vi "Disabled.vi"(7 "Robot Mode":T2=enum."Teleop Disabled", 10 "Match Info":T1={"Autonomous Elapsed Seconds"=0.0, "TeleOp Elapsed Seconds"=133.578, "Disabled Elapsed Seconds"=12.599, "Visited Autonomous"=FALSE, "Visited TeleOp"=TRUE, "Visited Disabled"=TRUE, "Autonomous Settings"={"Autonomous Style"=enum."Independent", "VI Refnum"=refnum}}, 11 "Call Context":T3=enum."Stop") -> ()   [LabVIEW 2012]
doc: "This VI is called each time a disabled packet is received from the DS. It is often used to prepare for the next robot mode, to calibrate sensors, etc."
uses:
  <vilib>/Rock Robotics/WPI/DriverStation/WPI_DriverStationDerivedRobotMode.ctl
  <vilib>/Rock Robotics/WPI/DriverStation/WPI_DriverStationRobotMode.ctl
  <vilib>/Rock Robotics/WPI/DriverStation/WPI_DriverStationMatch Info.ctl
  <vilib>/Rock Robotics/WPI/Solenoid/WPI_SolenoidValue.ctl
  Robot Global Data.vi
  <vilib>/Rock Robotics/WPI/Solenoid/WPI_SolenoidSetEnum.vi
panel:
  in  "Pitch Calib. Factor\nOLD ROBOT":dbl=-6.5
  in  "Encoder Codes\n Per Foot OLD Robot":u16=300
  in  "Feet/Second\n at FT OLD Robot":dbl=10.0
  in  "Encoder Codes\n Per Foot":u16=907
  in  "Feet/Second\n at Full Throttle":dbl=15.0
  in  "Pitch Calib. Factor\nNEW ROBOT":dbl=-1.7
  out "Loop Time":u32=23
  # "OLD"
  # "NEW"
  # "15"
  # "15   2011 Robot"
  # "907"
  # "300   2011 Robot"
  # "-0.5"
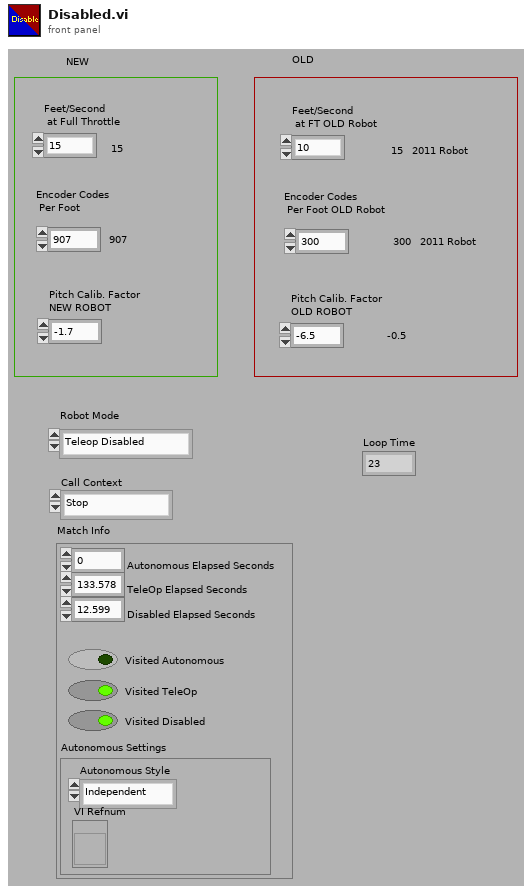
[diagram p1: front panel]
types:
  T1 = typedef "WPI_DriverStationMatch Info.ctl" = cluster{"Autonomous Elapsed Seconds":dbl, "TeleOp Elapsed Seconds":dbl, "Disabled Elapsed Seconds":dbl, "Visited Autonomous":bool, "Visited TeleOp":bool, "Visited Disabled":bool, "Autonomous Settings":cluster{"Autonomous Style":enum16{"Iterative", "Independent"}, "VI Refnum":refnum<vi>}}
  T2 = typedef "WPI_DriverStationRobotMode.ctl" = enum16{"Autonomous Disabled", "Autonomous Enabled", "Teleop Disabled", "Teleop Enabled", "Timeout", "Finish"}
  T3 = typedef "WPI_DriverStationDerivedRobotMode.ctl" = enum16{"Init", "Execute", "Stop"}
  T4 = typedef "WPI_SolenoidValue.ctl" = enum16{"Off", "On", "Forward", "Reverse"}
  T5 = typedef "WPI_SolenoidDevRef.ctl" = cluster{"DevStatus":errorcluster, "Solenoid Module":T6, "Forward Solenoid Channel":T7, "Reverse Solenoid Channel":T7}
  T6 = typedef "FPGA_TypedefSolenoidModule.ctl" = enum16{"Solenoid Module 1", "Solenoid Module 2"}
  T7 = typedef "WPI_SolenoidChannel.ctl" = enum8{"Solenoid 1", "Solenoid 2", "Solenoid 3", "Solenoid 4", "Solenoid 5", "Solenoid 6", "Solenoid 7", "Solenoid 8", "Invalid"}
  T8 = typedef "WPI_CounterDevRef.ctl" = cluster{"DevStatus":errorcluster, "CntIndex":T9}
  T9 = typedef "FPGA_CounterCtrSystemIndex.ctl" = enum8{"Ctr 0", "Ctr 1", "Ctr 2", "Ctr 3", "Ctr 4", "Ctr 5", "Ctr 6", "Ctr 7", "Invalid"}
  T10 = typedef "WPI_DigitalInputDevRef.ctl" = cluster{"DevStatus":errorcluster, "DIO Channel":T11, "Digital Module":T12}
  T11 = typedef "FPGA_DIOChannel.ctl" = enum8{"DIO 1", "DIO 2", "DIO 3", "DIO 4", "DIO 5", "DIO 6", "DIO 7", "DIO 8", "DIO 9", "DIO 10", "DIO 11", "DIO 12", "DIO 13", "DIO 14", "Invalid"}
  T12 = typedef "FPGA_TypedefDigitalModule.ctl" = enum16{"Digital Module 1", "Digital Module 2"}
  T13 = typedef "WPI_EncoderDevRef.ctl" = cluster{"DevStatus":errorcluster, "EncoderIndex":T14, "CounterIndex":T9, "DistancePerCount":dbl, "Decoding Type":T15}
  T14 = typedef "FPGA_EncoderIdx.ctl" = enum8{"Enc 0", "Enc 1", "Enc 2", "Enc 3", "Invalid"}
  T15 = typedef "WPI_EncoderType.ctl" = enum16{"1x", "2x", "4x"}
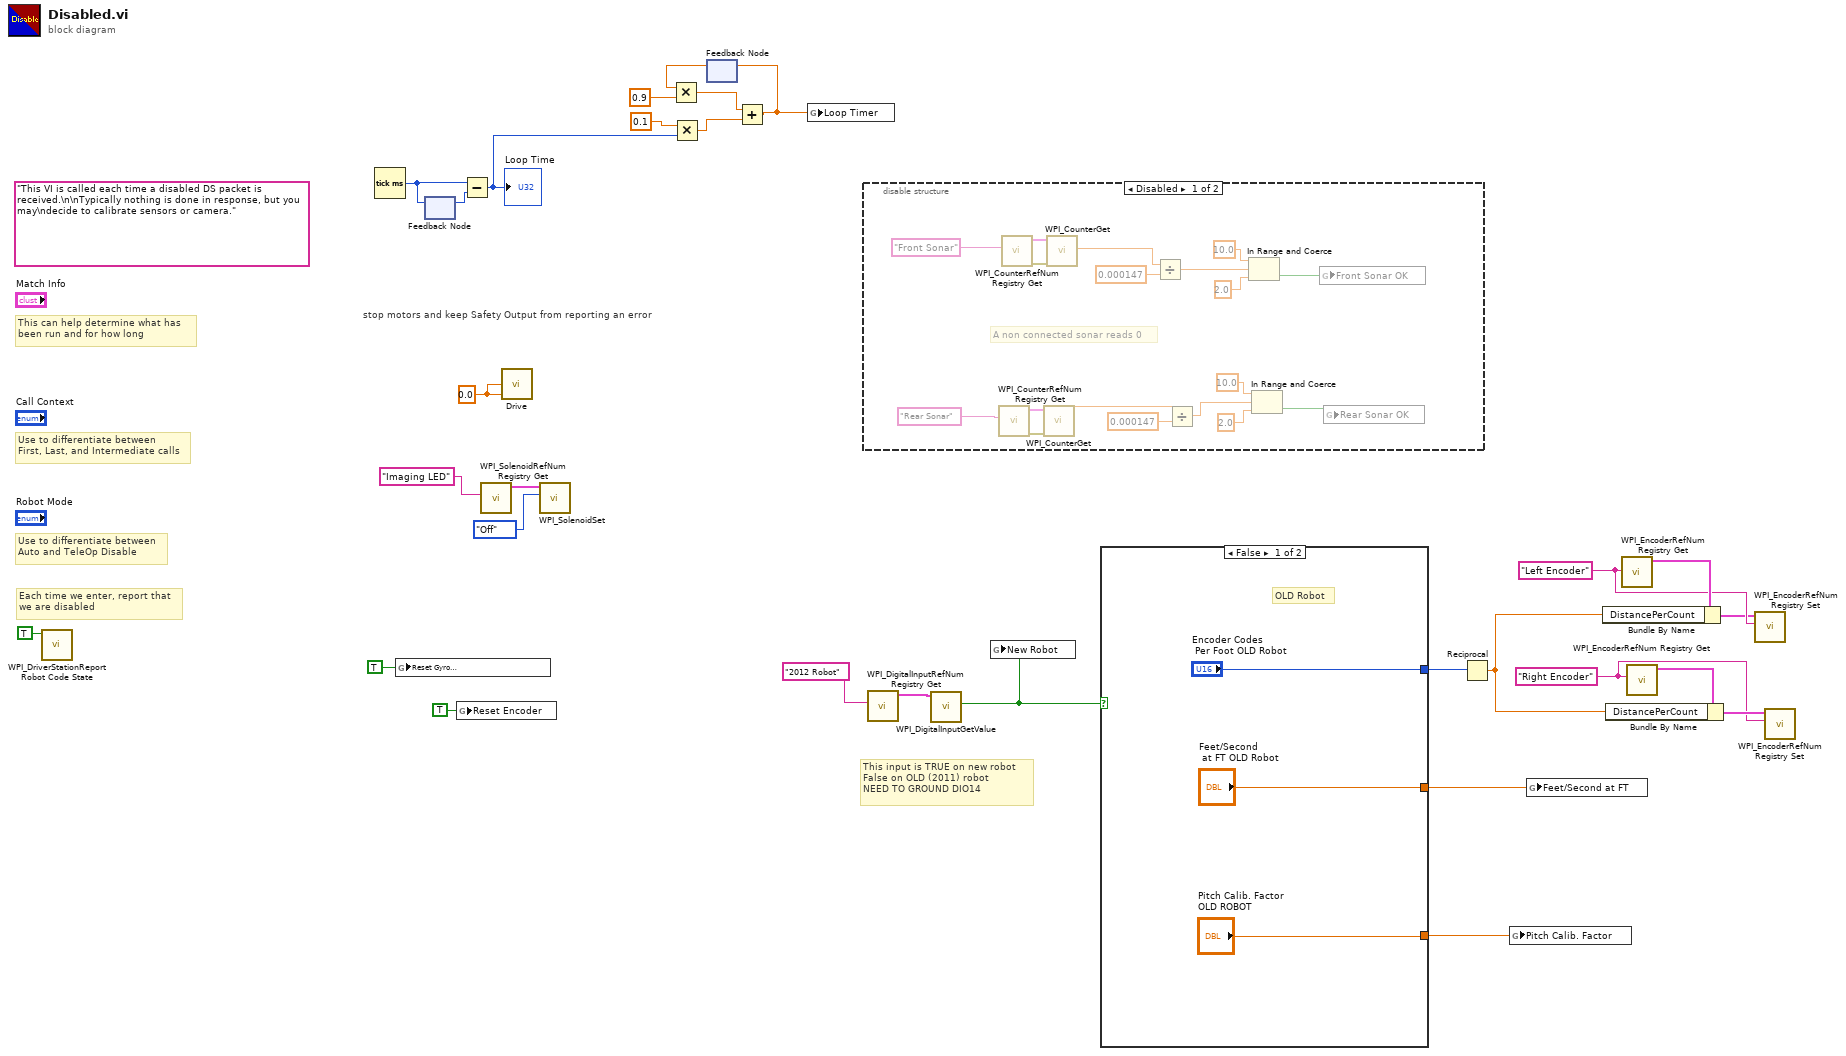
[diagram p0: block diagram]
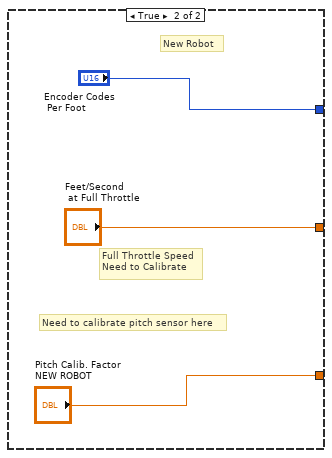
[diagram p3: hidden frame]
diagram:
  w3 = 0.0 ("Right Motor IN")
  w16 = "Right Encoder" ("refnum name")
  w21 = "Left Encoder" ("refnum name")
  (unwired) "This VI is called each time a disabled DS packet is received.\n\nTypically nothing is done in response, but you may\ndecide to calibrate sensors or camera."
  # "This input is TRUE on new robot\nFalse on OLD (2011) robot \nNEED TO GROUND DIO14"
  # "stop motors and keep Safety Output from reporting an error"
  # "Each time we enter, report that\nwe are disabled"
  # "Use to differentiate between\nFirst, Last, and Intermediate calls"
  # "This can help determine what has\nbeen run and for how long"
  # "Use to differentiate between\nAuto and TeleOp Disable"
  n1 = call <vilib>:"WPI_DriverStationReport Robot Code State.vi"("Disabled"=TRUE ("Autonomous")) -> ()  [unwired: 10 in, 1 out]
  n2 = Tick Count (ms)() -> (millisecond timer value=w27:u32)
  n3 = global write "Robot Global Data.vi" "Reset Gyro\nZero Position"(TRUE ("Reset Gyro\nZero Position")) -> ()
  n4 = feedback #1() -> (w28:u32)  [unwired: 1 in]
  n5 = feedback-in #1(w27) -> ()
  n6 = global write "Robot Global Data.vi" "Reset Encoder"(TRUE ("Reset Encoder")) -> ()
  n7 = Subtract(x=w27, y=w28) -> (x-y=w9:u32)
  "Loop Time" <- w9
  n8 = call <vilib>:"WPI_SolenoidRefNum Registry Get.vi"("refnum name"="Imaging LED") -> ("SolenoidDevRef"=w6:T5)  [unwired: 9 in, 1 out]
  n9 = call "Drive.vi"("Right Motor IN"=w3, "Left Motor IN"=w3) -> ()  [unwired: 3 in, 1 out]
  n10 = call-poly <vilib>:"WPI_SolenoidSet.vi"("Value"=WPI_SolenoidValue."Off", "SolenoidDevRef"=w6) -> ()  [unwired: 8 in, 2 out]
  n11 = Multiply(x=0.1, y=w9) -> (x*y=w11:dbl)
  n12 = feedback #2() -> (w13:dbl)  [unwired: 1 in]
  n13 = Multiply(x=w13, y=0.9) -> (x*y=w12:dbl)
  n14 = Add(x=w12, y=w11) -> (x+y=w15:dbl)
  n15 = feedback-in #2(w15) -> ()
  n16 = global write "Robot Global Data.vi" "Loop Timer"(w15) -> ()
  n17 = disable-structure shown="Disabled" {
    frame Disabled {
      # "A non connected sonar reads 0"
      n18 = call <vilib>:"WPI_CounterRefNum Registry Get.vi"("refnum name"="Rear Sonar") -> ("error out"=w43:errorcluster, "CounterDevRef"=w42:T8)  [unwired: 9 in]
      n19 = call <vilib>:"WPI_CounterRefNum Registry Get.vi"("refnum name"="Front Sonar") -> ("error out"=w47:errorcluster, "CounterDevRef"=w46:T8)  [unwired: 9 in]
      n20 = call <vilib>:"WPI_CounterGet.vi"("error in (no error)"=w43, "CounterDevRef in"=w42) -> ("Period (sec)"=w40:dbl)  [unwired: 4 in, 5 out]
      n21 = call <vilib>:"WPI_CounterGet.vi"("error in (no error)"=w47, "CounterDevRef in"=w46) -> ("Period (sec)"=w44:dbl)  [unwired: 4 in, 5 out]
      n22 = Divide(x=w44, y=0.000147 ("Scaling factor (s/in)")) -> (x/y=w34:dbl)
      n23 = Divide(x=w40, y=0.000147 ("Scaling factor (s/in)")) -> (x/y=w30:dbl)
      n24 = In Range and Coerce(upper limit=10.0 ("y"), x=w34, lower limit=2.0) -> (In Range?=w37:bool)  [unwired: 1 out]
      n25 = In Range and Coerce(upper limit=10.0 ("y"), x=w30, lower limit=2.0) -> (In Range?=w31:bool)  [unwired: 1 out]
      n26 = global write "Robot Global Data.vi" "Front Sonar OK"(w37) -> ()
      n27 = global write "Robot Global Data.vi" "Rear Sonar OK"(w31) -> ()
    }
    frame Enabled {
    }
  }
  n28 = call <vilib>:"WPI_DigitalInputRefNum Registry Get.vi"("refnum name"="2012 Robot") -> ("DigitalInputDevRef"=w25:T10)  [unwired: 9 in, 1 out]
  n29 = call <vilib>:"WPI_DigitalInputGetValue.vi"("DigitalInputDevRef"=w25) -> ("Value"=w8:bool)  [unwired: 8 in, 2 out]
  n30 = global write "Robot Global Data.vi" "New Robot"(w8) -> ()
  n31 = case shown="False" w8 {
    tunnel: ["Feet/Second\n at FT OLD Robot" "Feet/Second\n at Full Throttle"] -> w24
    tunnel: ["Encoder Codes\n Per Foot OLD Robot" "Encoder Codes\n Per Foot"] -> w23
    tunnel: ["Pitch Calib. Factor\nOLD ROBOT" "Pitch Calib. Factor\nNEW ROBOT"] -> w7
    frame False {
      # "OLD Robot"
    }
    frame True {
      # "Need to calibrate pitch sensor here"
      # "Full Throttle Speed\nNeed to Calibrate"
      # "New Robot"
    }
  }
  n32 = Reciprocal(x=w23) -> (1/x=w18:dbl)
  n33 = global write "Robot Global Data.vi" "Pitch Calib. Factor"(w7) -> ()
  n34 = global write "Robot Global Data.vi" "Feet/Second at FT"(w24) -> ()
  n35 = call <vilib>:"WPI_EncoderRefNum Registry Get.vi"("refnum name"=w21) -> ("EncoderDevRef"=w22:T13)  [unwired: 9 in, 1 out]
  n36 = Bundle By Name(cluster=w22, "DistancePerCount"=w18) -> (w20:T13)
  n37 = call <vilib>:"WPI_EncoderRefNum Registry Get.vi"("refnum name"=w16) -> ("EncoderDevRef"=w17:T13)  [unwired: 9 in, 1 out]
  n38 = Bundle By Name(cluster=w17, "DistancePerCount"=w18) -> (w19:T13)
  n39 = call <vilib>:"WPI_EncoderRefNum Registry Set.vi"("refnum name"=w21, "EncoderDevRef"=w20) -> ()  [unwired: 8 in, 2 out]
  n40 = call <vilib>:"WPI_EncoderRefNum Registry Set.vi"("refnum name"=w16, "EncoderDevRef"=w19) -> ()  [unwired: 8 in, 2 out]
